vi "_RemoveEvent (Index).vi"(8 "error in (no error)":errorcluster, 10 "Index":i32, 11 "EventBag in":refnum<class "EventBag.lvclass">) -> (0 "error out":errorcluster, 3 "EventBag out":refnum<class "EventBag.lvclass">)   [LabVIEW 2009, in "EventManagerLibrary.lvlib" / "EventBag.lvclass"]
uses:
  EventBag.lvclass
  EventBag.lvclass/EventBag.ctl
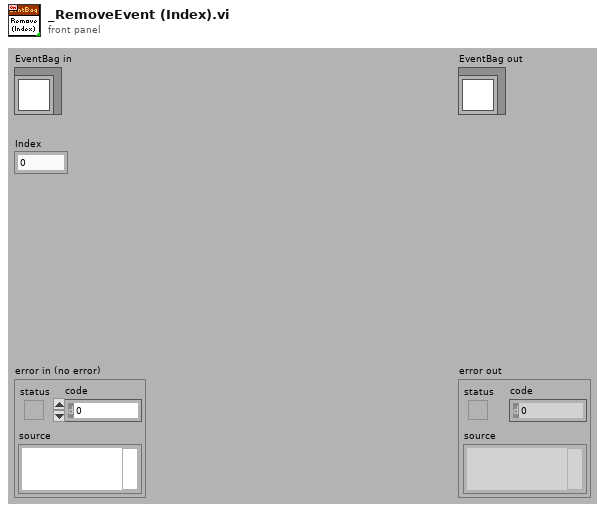
[diagram p1: front panel]
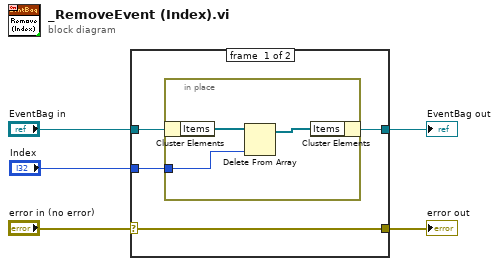
[diagram p0: block diagram]
diagram:
  n1 = case shown="No Error" "error in (no error)" {
    selector: "error in (no error)" -> [w9 w14]
    tunnel: [w9 w14] -> w4
    tunnel: [w7 w13] -> w2
    tunnel: "EventBag in" -> [w8 w13]
    tunnel: "Index" -> [w6 _]
    frame #0 {
      n2 = in-place {
        in-place-border: w6 -> [w11]
        n3 = in-place-cluster #1(w8) -> ("Items"=w12:refnum<class "Event.lvclass">[])
        n4 = Delete From Array(array=w12, index=w11) -> (array with subset deleted=w10:refnum<class "Event.lvclass">[])  [unwired: 1 in, 1 out]
        n5 = in-place-cluster #1("Items"=w10) -> (w7:refnum<class "EventBag.lvclass">)
      }
    }
    frame #1 {
    }
  }
  "error out" <- w4
  "EventBag out" <- w2
